vi "MainPC.vi"() -> ()   [LabVIEW 2025]
uses:
  type defs/state.ctl
  type defs/data.ctl
  <vilib>/vision/Image Controls.llb/IMAQ Image.ctl
  type defs/task.ctl
panel:
  in  "Mode":bool
  out "dup path":path
  out "image Analyed":T1(plugin-control)
  in  "SaveImage":bool
  out "image display":T1(plugin-control)
  in  "Stop":bool
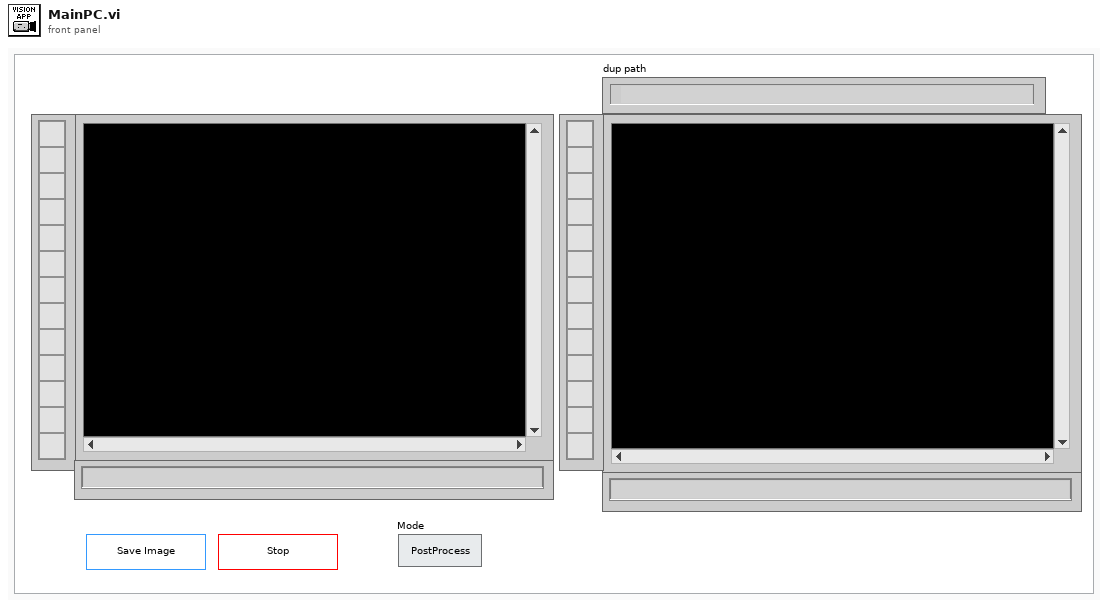
[diagram p1: front panel]
types:
  T1 = typedef "IMAQ Image.ctl" = refnum<image>
  T2 = typedef "data.ctl" = cluster{"save image":bool, "qsm":cluster{"Webcam image ref":T1, "Analyzed image ref":T1, "Stop webcam":bool}, "R-Pixel":dbl}
  T3 = typedef "state.ctl" = enum16{"(qsm) schedule", "(qsm) initialize", "(qsm) release", "(qsm) clean up", "(qsm) shutdown", "(HW) initialize", "((HW)) clean up", "((HW)) update ports", "(image) get", "(image) analyze", "(image) overlay", "(image) show", "save image", "state A", "state B", "state C", "state D", "state E", "state F", "state G", "state H"}
  T4 = cluster{"Desired Font (Application)":enum16{"User-specified Font", "Application Font", "System Font", "Dialog Font"}, "[User-specified Font]":cluster{"Font Name":string, "Size":i16, "Strikeout?":bool, "Italic?":bool, "Underline?":bool, "Outline?":bool, "Shadow?":bool, "Bold?":bool, "Rotation Angle":dbl}, "Horizontal Alignment":i16, "Vertical Alignment":i16}
  T5 = typedef "task.ctl" = T3[]
  T6 = cluster{"Center (Pixels)":cluster{"X":sgl, "Y":sgl}, "Radius (Pixels)":dbl, "Center (Real-World)":cluster{"X":sgl, "Y":sgl}, "Radius (Real-World)":dbl, "Roundness (Real-World)":dbl, "Average Strength":dbl, "Average SNR (dB)":dbl}
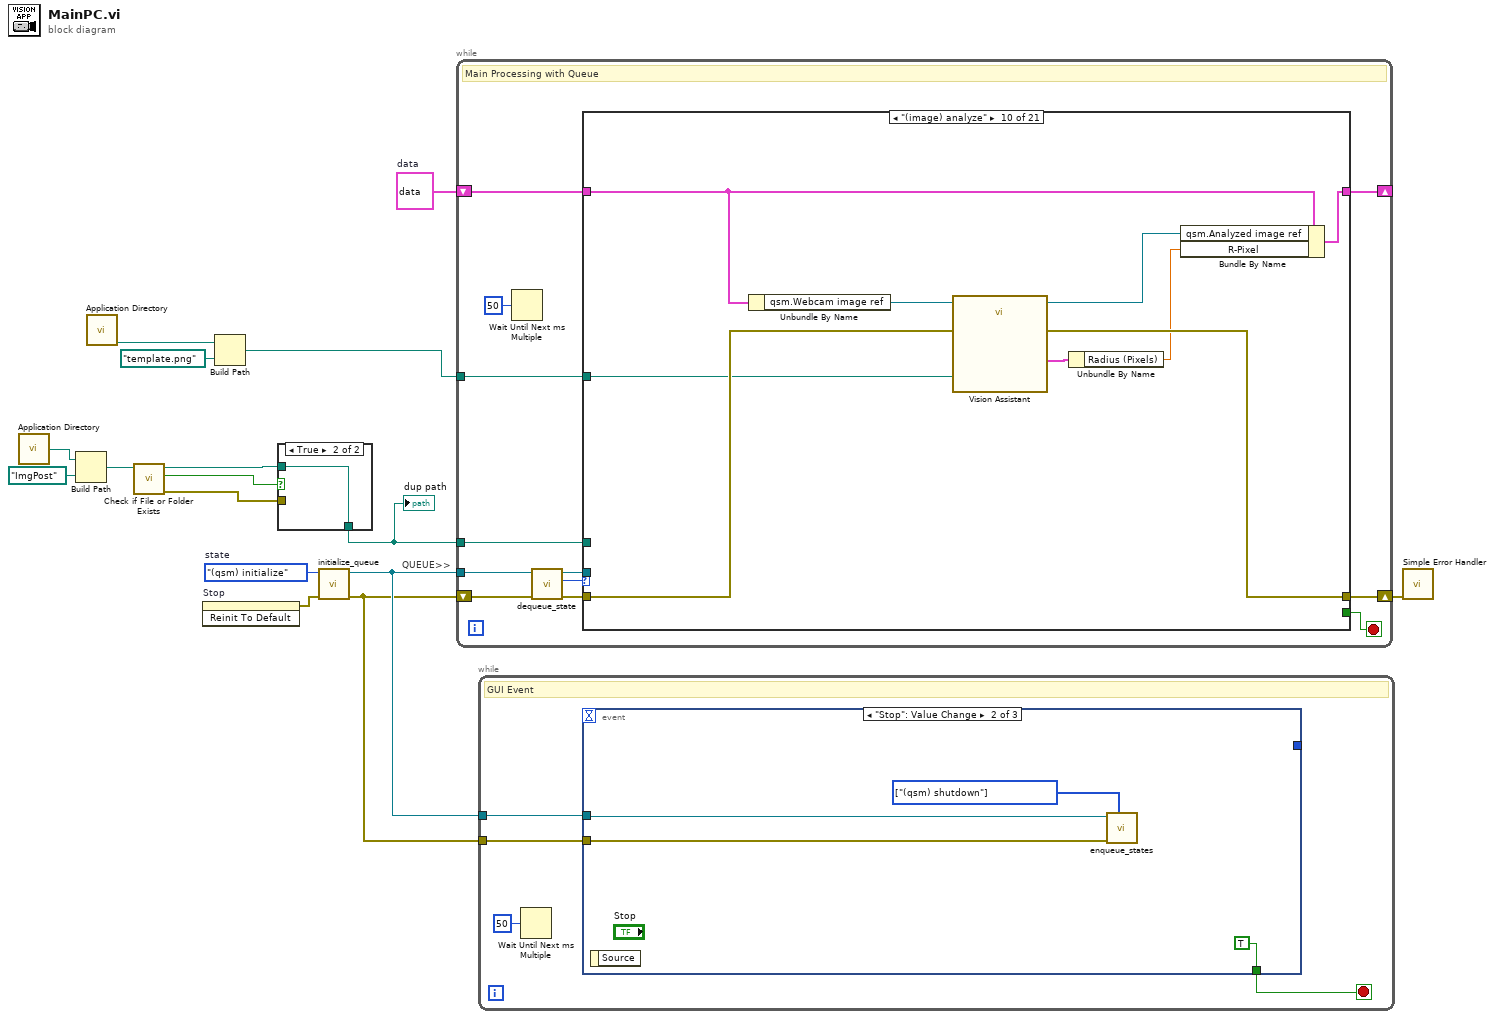
[diagram p0: block diagram]
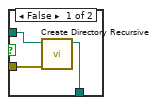
[diagram p2: hidden frame]
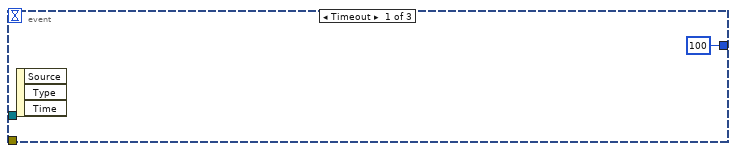
[diagram p3: hidden frame]
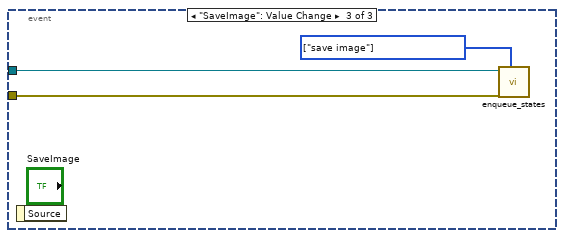
[diagram p4: hidden frame]
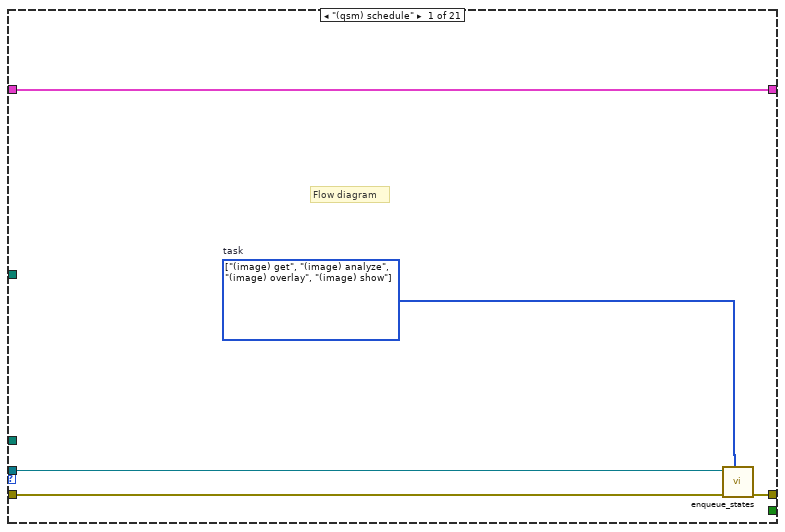
[diagram p5: hidden frame]
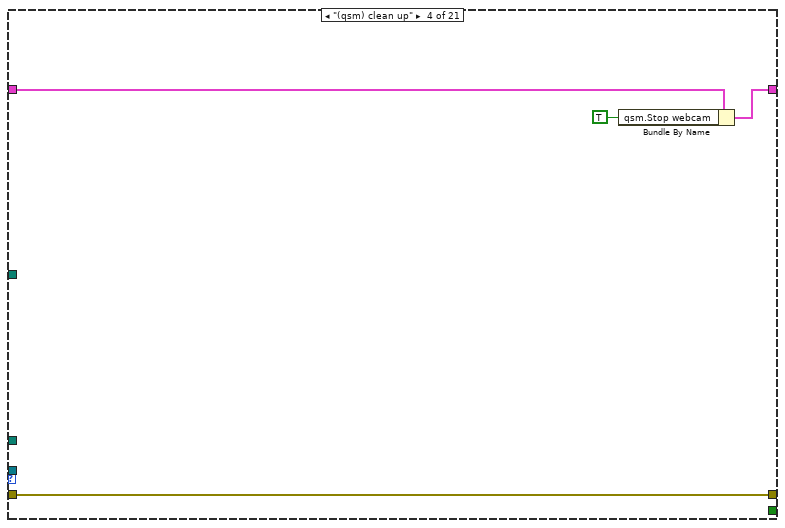
[diagram p8: hidden frame]
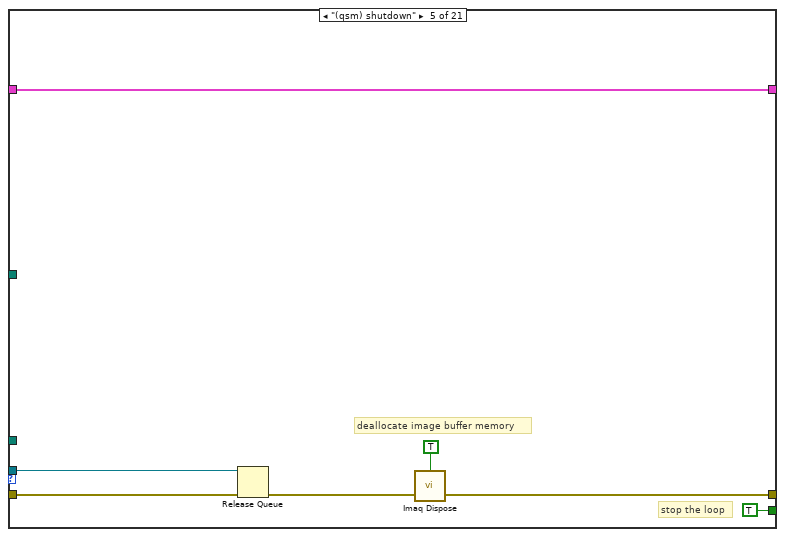
[diagram p9: hidden frame]
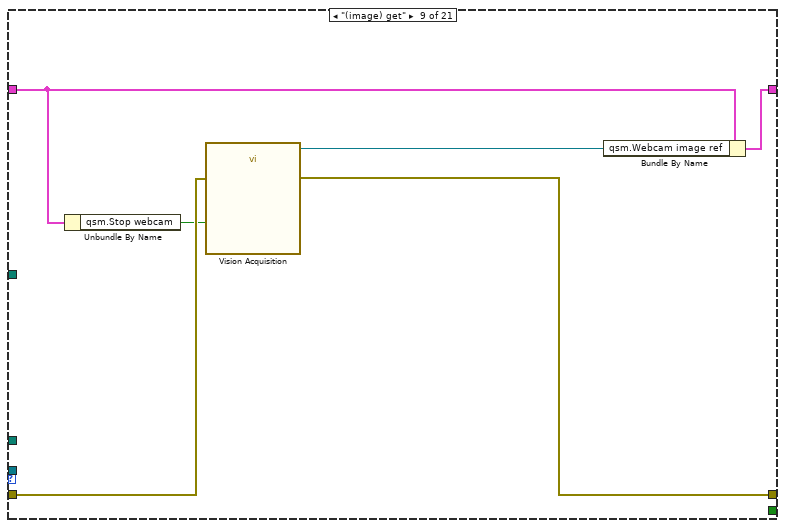
[diagram p13: hidden frame]
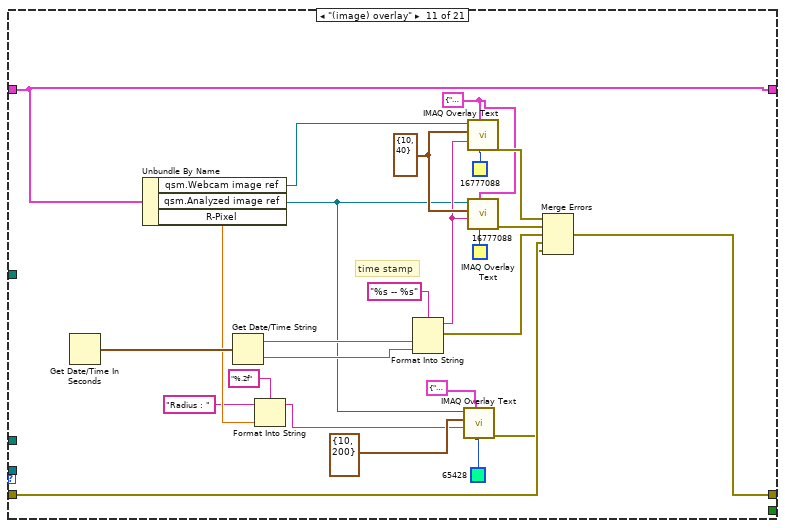
[diagram p14: hidden frame]
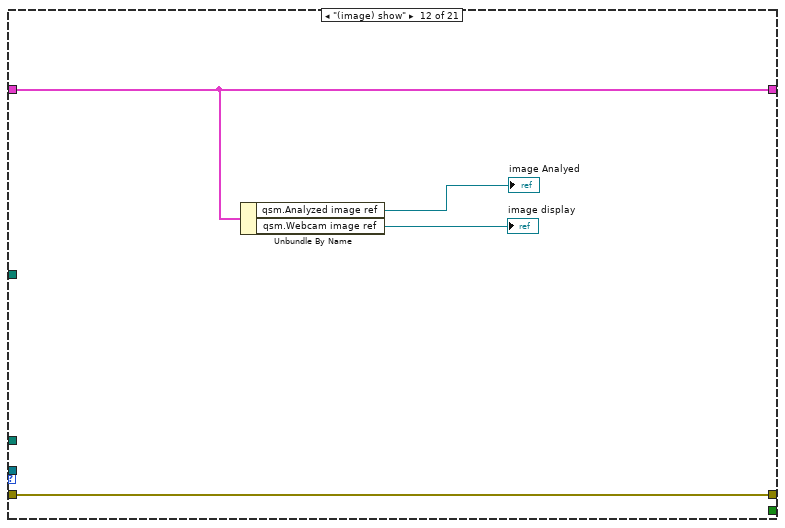
[diagram p15: hidden frame]
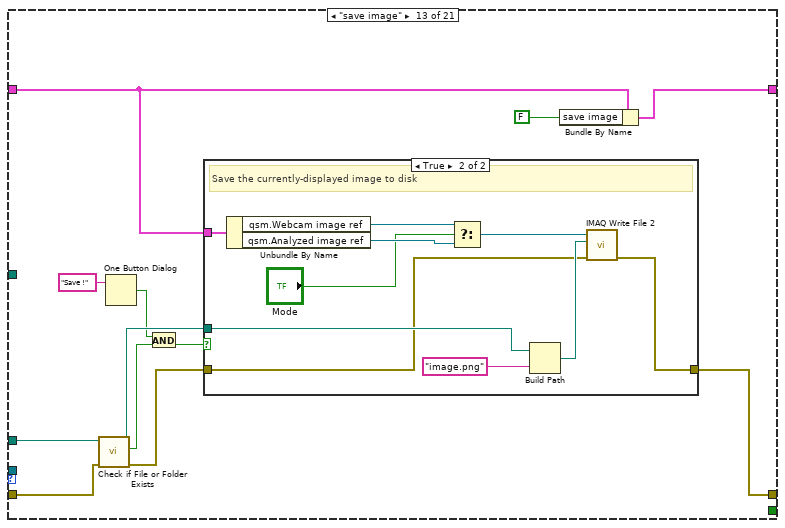
[diagram p16: hidden frame]
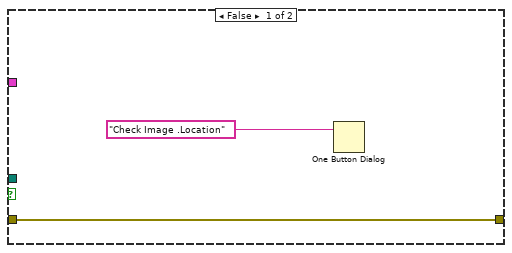
[diagram p17: hidden frame]
diagram:
  w15 = T2 {"save image"=FALSE, "qsm"={"Webcam image ref"=refnum, "Analyzed image ref"=refnum, "Stop webcam"=FALSE}, "R-Pixel"=0.0}  # data
  w13 = state."(qsm) initialize"  # state
  # "QUEUE>>"
  n1 = call <vilib>:"Application Directory.vi"() -> ("Application Directory"=w10:path)
  n2 = Build Path(base path=w10, name or relative path=path "ImgPost") -> (appended path=w8:path)
  n3 = call <vilib>:"Application Directory.vi"() -> ("Application Directory"=w3:path)
  n4 = call <vilib>:"Check if File or Folder Exists.vi"("path"=w8) -> ("error out"=w5:errorcluster, "file or folder exists?"=w7:bool, "dup path"=w6:path)  [unwired: 8 in]
  n5 = invoke on="Stop" class="Bool" method="Reinit To Default"() -> (error out=w14:errorcluster)  [unwired: 3 in, 2 out]
  n6 = Build Path(base path=w3, name or relative path=path "template.png") -> (appended path=w2:path)
  n7 = case shown="True" w7 {
    tunnel: w6 -> [w19 w20]
    tunnel: w5 -> [w18 _]
    tunnel: [w17 w20] -> w4
    frame False {
      n8 = call <vilib>:"Create Directory Recursive.vi"("error in (no error)"=w18, "directory"=w19) -> ("directory copy"=w17:path)  [unwired: 3 in, 2 out]
    }
    frame True {
    }
  }
  "dup path" <- w4
  n9 = call "initialize_queue.vi"("error in (no error)"=w14, "state"=w13) -> ("error out"=w11:errorcluster, "queue out"=w12:refnum<queue>)  [unwired: 8 in]
  n10 = while {
    shift-right: [w32] -> w16
    shift-left: w11 -> [w26]
    tunnel: w12 -> [w27]
    shift-right: [w30] -> _
    shift-left: w15 -> [w31]
    tunnel: w4 -> [w22]
    tunnel: w2 -> [w21]
    stop <- w29 stop-if-true
    # "Main Processing with Queue"
    n11 = Wait Until Next ms Multiple(millisecond multiple=u32 50) -> ()  [unwired: 1 out]
    n12 = call "dequeue_state.vi"("error in (no error)"=w26, "queue in"=w27) -> ("error out"=w28:errorcluster, "state"=w23:T3, "queue out"=w25:refnum<queue>)  [unwired: 7 in]
    n13 = case shown="\"(image) analyze\"" w23 {
      tunnel: w28 -> [w35 w39 w40 w42 w51 w53 w55 w57 w64 w69 w84 w101 w111 w128 w130 w132 w134 w136 w137 w139 w142]
      tunnel: w25 -> [w36 _ _ _ w50 _ _ _ _ _ _ _ _ _ _ _ _ _ _ _ _]
      tunnel: [w37 w39 w40 w42 w46 w53 w55 w57 w59 w68 w93 w101 w110 w128 w130 w132 w134 w136 w137 w139 w142] -> w32
      tunnel: w31 -> [w34 w38 w41 w44 w49 w54 w56 w58 w62 w73 w85 w102 w114 w127 w129 w131 w133 w135 w138 w140 w141]
      tunnel: [w34 w38 w41 w43 w49 w54 w56 w58 w63 w72 w85 w102 w113 w127 w129 w131 w133 w135 w138 w140 w141] -> w30
      tunnel: [_ _ _ _ TRUE _ _ _ _ _ _ _ _ _ _ _ _ _ _ _ _] -> w29
      tunnel: w22 -> [_ _ _ _ _ _ _ _ _ _ _ _ w107 _ _ _ _ _ _ _ _]
      tunnel: w21 -> [_ _ _ _ _ _ _ _ _ w65 _ _ _ _ _ _ _ _ _ _ _]
      frame "(qsm) schedule" {
        w33 = T5 [enum."(image) get", enum."(image) analyze", enum."(image) overlay", enum."(image) show"] items=["(qsm) schedule", "(qsm) initialize", "(qsm) release", "(qsm) clean up", "(qsm) shutdown", "(HW) initialize", "((HW)) clean up", "((HW)) update ports", "(image) get", "(image) analyze", "(image) overlay", "(image) show", "save image", "state A", "state B", "state C", "state D", "state E", "state F", "state G", "state H"]  # task
        # "Flow diagram"
        # "Startup ... Schedule"
        n14 = call "enqueue_states.vi"("task"=w33, "error in"=w35, "queue in"=w36) -> ("error out"=w37:errorcluster)  [unwired: 7 in, 1 out]
      }
      frame "(qsm) initialize" {
      }
      frame "(qsm) release" {
        # "Release all front-panel action buttons."
      }
      frame "(qsm) clean up" {
        # "Clean up -- Set the \"Stop webcam flag\" and perform other necessary clean-up actions."
        n15 = Bundle By Name(cluster=w44, "qsm.Stop webcam"=TRUE) -> (w43:T2)
      }
      frame "(qsm) shutdown" {
        # "deallocate image buffer memory"
        # "stop the loop"
        # "Shutdown -- Release the state queue, free all image buffer memory, and stop the while-loop structure."
        n16 = Release Queue(queue=w50, error in (no error)=w51) -> (error out=w47:errorcluster)  [unwired: 1 in, 2 out]
        n17 = call "Imaq Dispose"("All Images? (No)"=TRUE, "error in (no error)"=w47) -> ("error out"=w46:errorcluster)  [unwired: 4 in]
      }
      frame "(HW) initialize" {
      }
      frame "((HW)) clean up" {
      }
      frame "((HW)) update ports" {
        # "set the flag"
        # "Update ports (myRIO) -- Read and write onboard devices and external peripherals."
      }
      frame "(image) get" {
        # "Get image -- Retrieve a single webcam image frame and optionally flip the image right side up."
        n18 = Unbundle By Name(w62) -> ("qsm.Stop webcam"=w61:bool)
        n19 = call "Vision Acquisition"("Stop (F)"=w61, "error in"=w64) -> ("Image Out"=w60:T1, "error out"=w59:errorcluster)  [unwired: 23 in, 1 out]
        n20 = Bundle By Name(cluster=w62, "qsm.Webcam image ref"=w60) -> (w63:T2)
      }
      frame "(image) analyze" {
        n21 = Unbundle By Name "Unbundle By Name"(w73) -> ("qsm.Webcam image ref"=w71:T1)
        n22 = call "Vision Assistant"("Image In"=w71, "Template File Path (Pattern Matching 1)"=w65, "error in"=w69) -> ("Image Out"=w70:T1, "Fitted Circle (Find Circular Edge 1)"=w67:T6, "error out"=w68:errorcluster)  [unwired: 22 in]
        n23 = Unbundle By Name(w67) -> ("Radius (Pixels)"=w66:dbl)
        n24 = Bundle By Name "Bundle By Name"(cluster=w73, "qsm.Analyzed image ref"=w70, "R-Pixel"=w66) -> (w72:T2)
      }
      frame "(image) overlay" {
        w83 = T4 {"Desired Font (Application)"=enum."Application Font", "[User-specified Font]"={"Font Name"="", "Size"=18, "Strikeout?"=FALSE, "Italic?"=FALSE, "Underline?"=FALSE, "Outline?"=FALSE, "Shadow?"=FALSE, "Bold?"=FALSE, "Rotation Angle"=0.0}, "Horizontal Alignment"=0, "Vertical Alignment"=0} ("Font, Size & Style")
        w95 = cluster{"X":i32, "Y":i32} {"X"=10, "Y"=40} ("Origin")
        # "time stamp"
        n25 = Get Date/Time In Seconds() -> (seconds since 1Jan1904=w89:timestamp)
        n26 = Unbundle By Name "Unbundle By Name"(w85) -> ("qsm.Webcam image ref"=w96:T1, "qsm.Analyzed image ref"=w82:T1, "R-Pixel"=w80:dbl)
        n27 = Get Date/Time String(seconds (now)=w89) -> (date string=w88:string, time string=w87:string)  [unwired: 2 in]
        n28 = Format Into String(format string="%.2f", initial string="Radius : ", w80) -> (resulting string=w79:string)  [unwired: 1 in, 1 out]
        n29 = Format Into String "Format Into String"(format string="%s -- %s", w88, w87) -> (resulting string=w90:string, error out=w86:errorcluster)  [unwired: 2 in]
        n30 = call "IMAQ Overlay Text"("Text Color (black)"=u32 65428, "Font, Size & Style"=T4 {"Desired Font (Application)"=enum."Application Font", "[User-specified Font]"={"Font Name"="", "Size"=50, "Strikeout?"=FALSE, "Italic?"=FALSE, "Underline?"=FALSE, "Outline?"=FALSE, "Shadow?"=FALSE, "Bold?"=FALSE, "Rotation Angle"=0.0}, "Horizontal Alignment"=0, "Vertical Alignment"=0}, "String"=w79, "Origin"=cluster{"X":i32, "Y":i32} {"X"=10, "Y"=200}, "Image"=w82) -> ("error out"=w78:errorcluster)  [unwired: 5 in, 1 out]
        n31 = call "IMAQ Overlay Text"("Text Color (black)"=u32 16777088, "Font, Size & Style"=w83, "String"=w90, "Origin"=w95, "Image"=w96) -> ("error out"=w92:errorcluster)  [unwired: 5 in, 1 out]
        n32 = call "IMAQ Overlay Text"("Text Color (black)"=u32 16777088, "Font, Size & Style"=w83, "String"=w90, "Origin"=w95, "Image"=w82) -> ("error out"=w94:errorcluster)  [unwired: 5 in, 1 out]
        n33 = Merge Errors "Merge Errors"(w92, w94, w86, w84, w78) -> (w93:errorcluster)
      }
      frame "(image) show" {
        # "Show image -- Select from among the available image buffers to show on the main image display; use a selector tree or case structure."
        n34 = Unbundle By Name "Unbundle By Name"(w102) -> ("qsm.Analyzed image ref"=→"image Analyed":T1, "qsm.Webcam image ref"=→"image display":T1)
      }
      frame "save image" {
        # "Save image (example of an application-specific state) -- Save either the original webcam image or the analyzed image with overlay to a PNG file on the USB flash drive connected to myRIO."
        n35 = call <vilib>:"Check if File or Folder Exists.vi"("error in (no error)"=w111, "path"=w107) -> ("error out"=w108:errorcluster, "file or folder exists?"=w109:bool, "dup path"=w106:path)  [unwired: 7 in]
        n36 = One Button Dialog(message="Save !") -> (true=w103:bool)  [unwired: 1 in]
        n37 = And(x=w103, y=w109) -> (x .and. y?=w104:bool)
        n38 = case shown="True" w104 {
          tunnel: w114 -> [_ w125]
          tunnel: [w115 w123] -> w110
          tunnel: w108 -> [w115 w117]
          tunnel: w106 -> [_ w122]
          frame False {
            n39 = One Button Dialog(message="Check Image .Location") -> ()  [unwired: 1 in, 1 out]
          }
          frame True {
            # "Save the currently-displayed image to disk"
            n40 = Unbundle By Name(w125) -> ("qsm.Webcam image ref"=w121:T1, "qsm.Analyzed image ref"=w120:T1)
            n41 = Select(t=w121, s="Mode", f=w120) -> (s? t:f=w119:T1)
            n42 = Build Path(base path=w122, name or relative path="image.png") -> (appended path=w126:path)
            n43 = call-poly "IMAQ Write File 2"("error in (no error)"=w117, "File Path"=w126, "Image"=w119) -> ("error out"=w123:errorcluster)  [unwired: 7 in, 1 out]
          }
        }
        n44 = Bundle By Name(cluster=w114, "save image"=FALSE) -> (w113:T2)
      }
      frame "state A" {
        # "Expansion State A"
      }
      frame "state B" {
        # "Expansion State B"
      }
      frame "state C" {
        # "Expansion State C"
      }
      frame "state D" {
        # "Expansion State D"
      }
      frame "state E" {
        # "Expansion State E"
      }
      frame "state F" {
        # "Expansion State F"
      }
      frame "state G" {
        # "Expansion State G"
      }
      frame "state H" {
        # "Expansion State H"
      }
    }
  }
  n45 = while {
    tunnel: w12 -> [w146]
    tunnel: w11 -> [w145]
    stop <- w144 stop-if-true
    # "GUI Event"
    n46 = Wait Until Next ms Multiple(millisecond multiple=u32 50) -> ()  [unwired: 1 out]
    n47 = event shown="[1] \"Stop\": Value Change" {
      selector: _ -> [_ _ _]
      dyn-events: _ -> [_ _ _]
      timeout: _ -> [_ _ _]
      tunnel: w146 -> [_ w151 w153]
      tunnel: w145 -> [_ w150 w152]
      tunnel: [_ TRUE _] -> w144
      tunnel: [100 _ _] -> _
      event Timeout {
        n48 = event-data() -> ()  [unwired: 1 in, 3 out]
      }
      event "Stop": Value Change {
        w149 = T5 [enum."(qsm) shutdown"] items=["(qsm) schedule", "(qsm) initialize", "(qsm) release", "(qsm) clean up", "(qsm) shutdown", "(HW) initialize", "((HW)) clean up", "((HW)) update ports", "(image) get", "(image) analyze", "(image) overlay", "(image) show", "save image", "state A", "state B", "state C", "state D", "state E", "state F", "state G", "state H"] ("task")
        n49 = event-data() -> ()  [unwired: 1 in, 1 out]
        n50 = call "enqueue_states.vi"("task"=w149, "error in"=w150, "queue in"=w151) -> ()  [unwired: 7 in, 2 out]
      }
      event "SaveImage": Value Change {
        w154 = T5 [enum."save image"] items=["(qsm) schedule", "(qsm) initialize", "(qsm) release", "(qsm) clean up", "(qsm) shutdown", "(HW) initialize", "((HW)) clean up", "((HW)) update ports", "(image) get", "(image) analyze", "(image) overlay", "(image) show", "save image", "state A", "state B", "state C", "state D", "state E", "state F", "state G", "state H"] ("task")
        n51 = event-data() -> ()  [unwired: 1 in, 1 out]
        n52 = call "enqueue_states.vi"("task"=w154, "error in"=w152, "queue in"=w153) -> ()  [unwired: 7 in, 2 out]
      }
    }
  }
  n53 = call <vilib>:"Simple Error Handler.vi"("error in (no error)"=w16) -> ()  [unwired: 4 in, 5 out]
